vi "move to target point.vi"(2 "PIS Close":bool, 8 "precision of nodes":i32=6, 9 "Litho Speed":dbl=5e-07 format="%#_6pm/s", 10 "Z SetPoint":dbl format="%#_6p", 11 "Target Point\n(  x      ,       y   )":dbl[](array[numeric])=[-5e-06, -5e-06] min=-4.5e-05 max=4.5e-05 step=1e-09 format="%#_6pm") -> ()   [LabVIEW 2013]
uses:
  simulator/Global Variables.vi
  Cypher XY LVDT Parameters.vi
panel:
  in  "?":bool
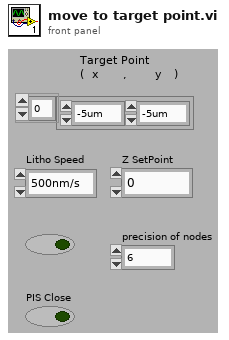
[diagram p1: front panel]
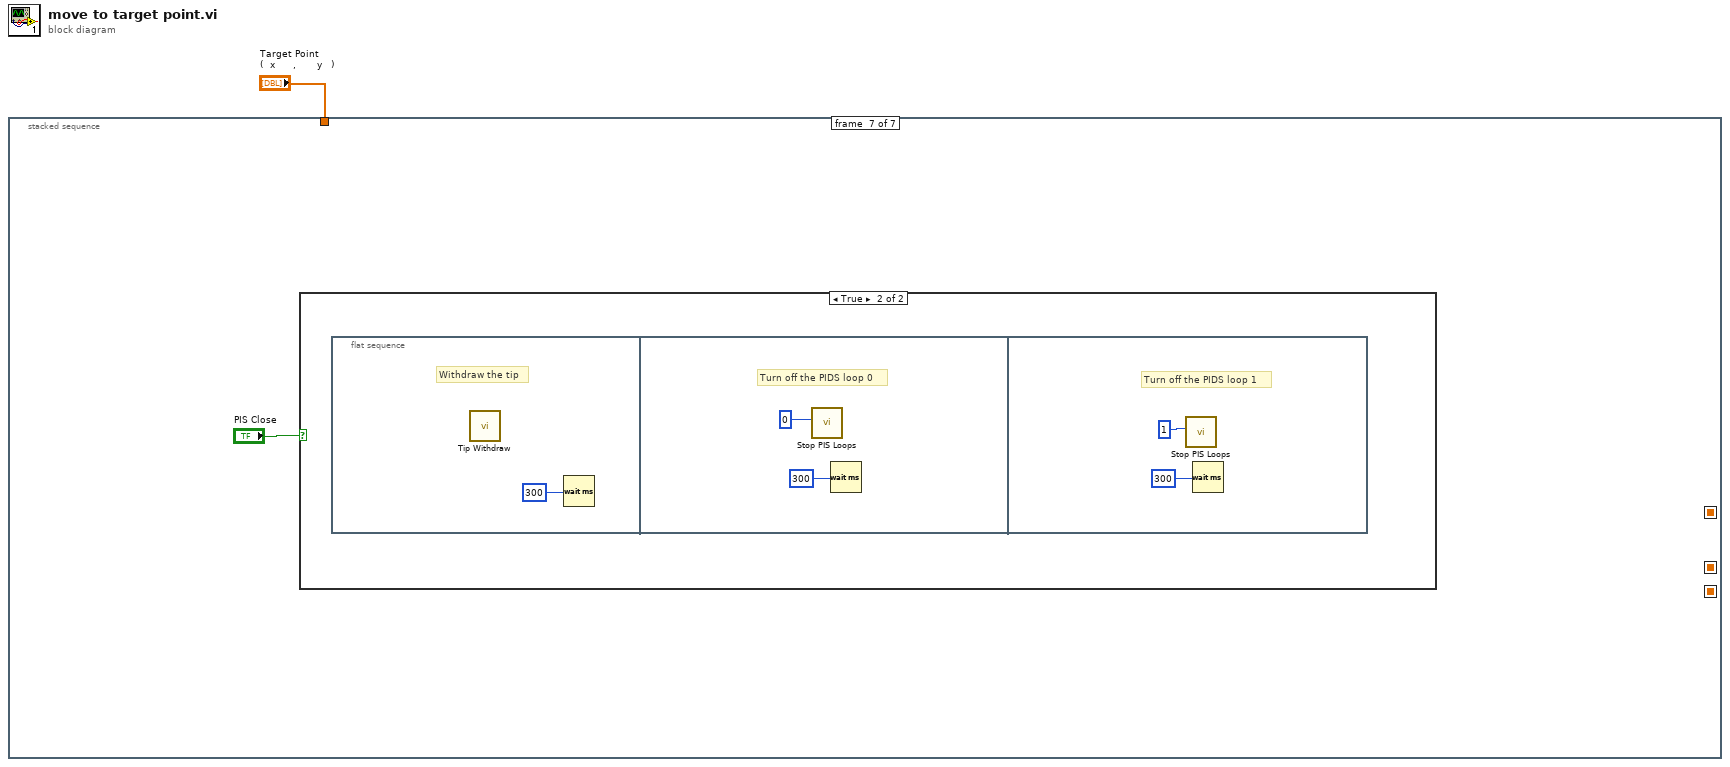
[diagram p0: block diagram]
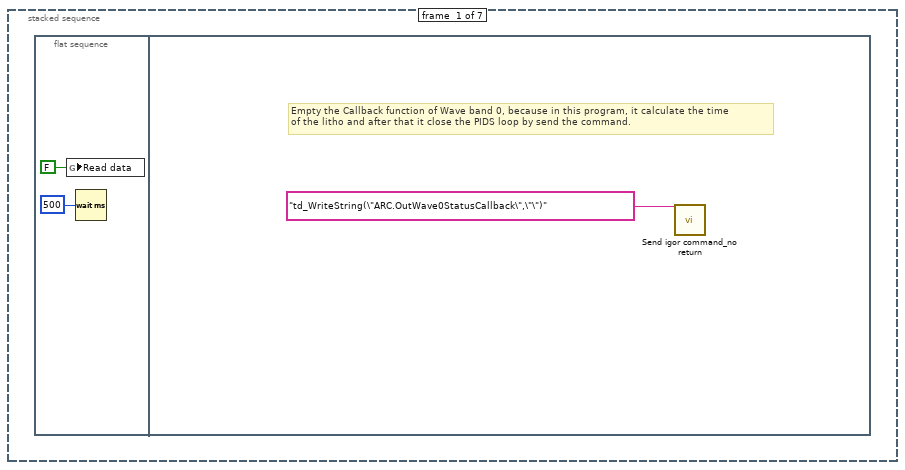
[diagram p2: hidden frame]
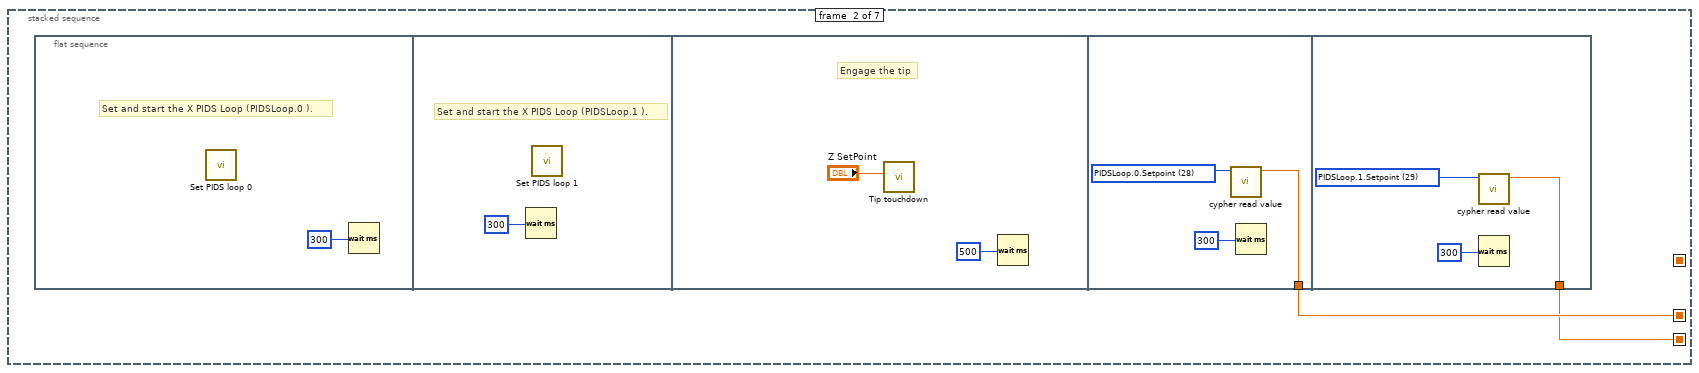
[diagram p3: hidden frame]
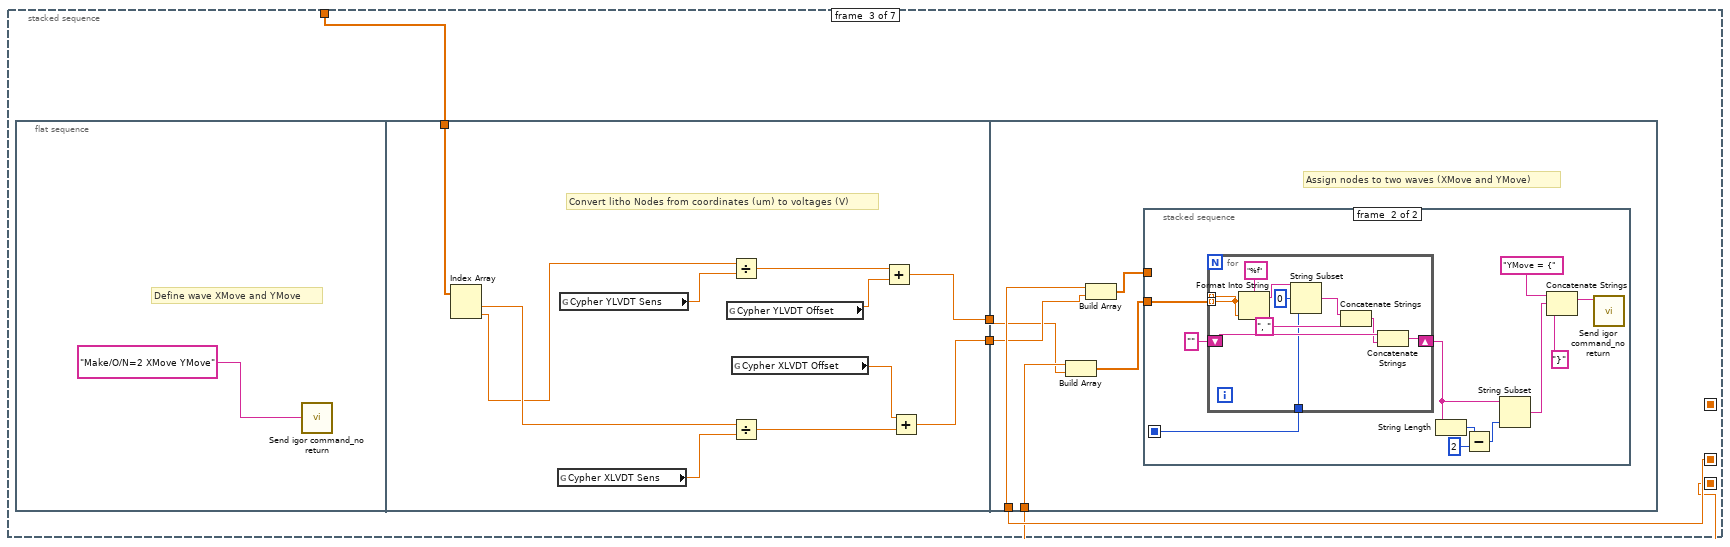
[diagram p4: hidden frame]
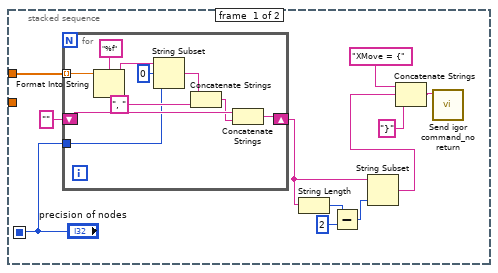
[diagram p5: hidden frame]
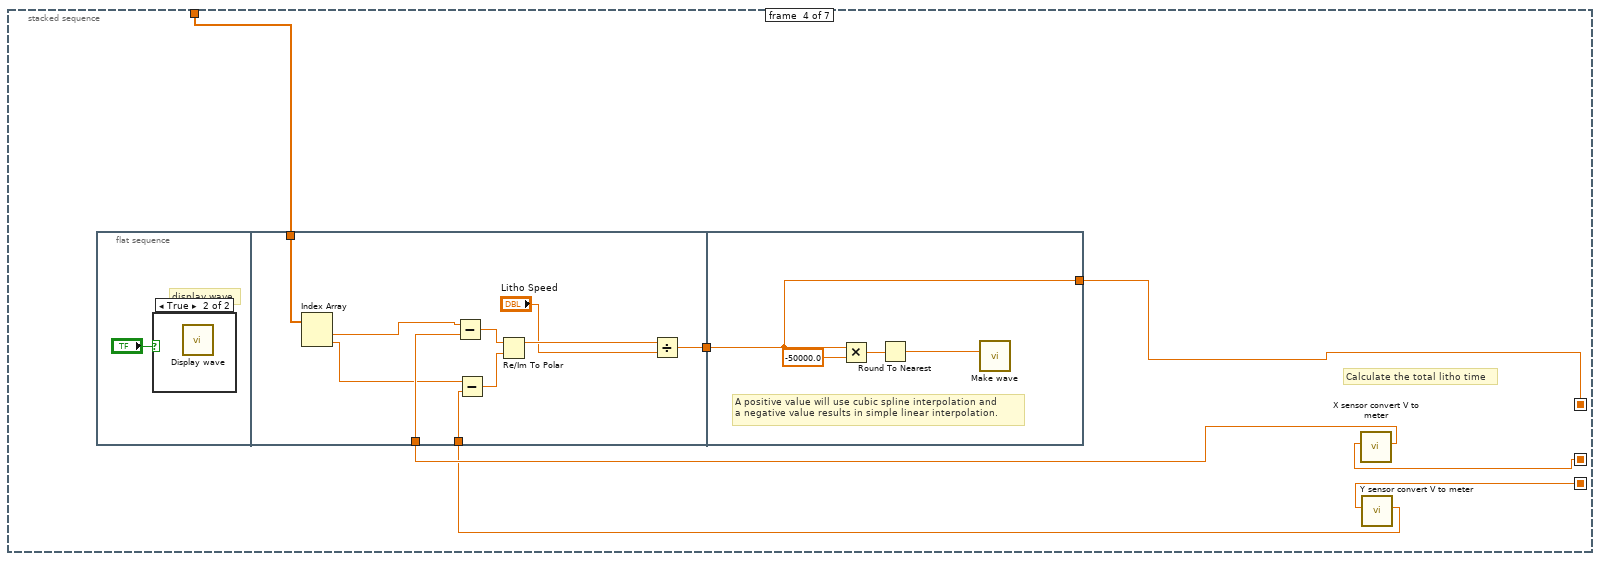
[diagram p6: hidden frame]
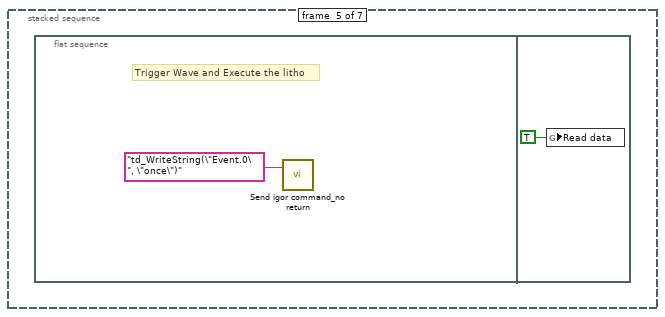
[diagram p8: hidden frame]
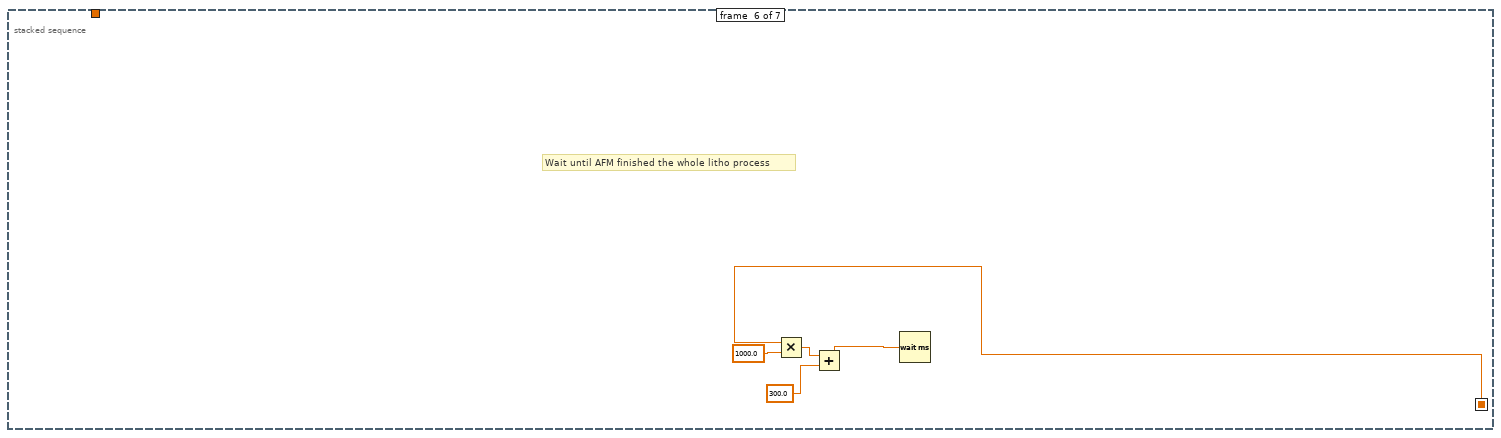
[diagram p9: hidden frame]
diagram:
  n1 = stacked-sequence {
    seq-local: [_ _ _ w87 _ _ _] -> [_ _ _ _ _ w109 _]
    seq-local: [_ w6 _ _ _ _ _] -> [_ _ w18 w86 _ _ _]
    seq-local: [_ w5 _ _ _ _ _] -> [_ _ w17 w85 _ _ _]
    tunnel: "Target Point\n(  x      ,       y   )" -> [_ _ w19 w84 _ _ _]
    frame #0 {
      n2 = flat-sequence {
        frame #0 {
          n3 = global write "Global Variables.vi" "Read data"(FALSE ("Read data")) -> ()
          n4 = Wait (ms)(milliseconds to wait=u32 500) -> ()  [unwired: 1 out]
        }
        frame #1 {
          # "Empty the Callback function of Wave band 0, because in this program, it calculate the time \nof the litho and after that it close the PIDS loop by send the command."
          n5 = call "Send igor command_no return.vi"("Command"="td_WriteString(\"ARC.OutWave0StatusCallback\",\"\")") -> ()  [unwired: 11 out]
        }
      }
    }
    frame #1 {
      n6 = flat-sequence {
        tunnel: [w12] -> w6
        tunnel: [w15] -> w5
        frame #0 {
          # "Set and start the X PIDS Loop (PIDSLoop.0 )."
          n7 = call "Set PIDS loop 0.vi"() -> ()  [unwired: 12 in]
          n8 = Wait (ms)(milliseconds to wait=u32 300) -> ()  [unwired: 1 out]
        }
        frame #1 {
          # "Set and start the X PIDS Loop (PIDSLoop.1 )."
          n9 = Wait (ms)(milliseconds to wait=u32 300) -> ()  [unwired: 1 out]
          n10 = call "Set PIDS loop 1.vi"() -> ()  [unwired: 12 in]
        }
        frame #2 {
          # "Engage the tip"
          n11 = call "Tip touchdown.vi"("Z SetPoint"="Z SetPoint") -> ()  [unwired: 11 out]
          n12 = Wait (ms)(milliseconds to wait=u32 500) -> ()  [unwired: 1 out]
        }
        frame #3 {
          w13 = u16 28 items=["XSensor", "YSensor", "ZSensor", "InA", "InB", "InFast", "In_Amplitude1", "In_Amplitude2", "In_Phase1", "In_Phase2", "PiezoX", "PiezoY", "PiezoZ", "OutA", "OutB", "OutC", "DDS_Frequency1", "DDS_Frequency2", "DDS_Amplitude1", "DDS_Amplitude2", "DDS_DCOffset", "Laser_Sum", "Laser_Difference", "Laser_Lateral", "XLVDT Sensitivity", "YLVDT Sensitivity", "XLVDT Offset", "YLVDT Offset", "PIDSLoop.0.Setpoint", "PIDSLoop.1.Setpoint"] ("Input")
          n13 = call "cypher read value.vi"("Input"=w13) -> ("Result"=w12:dbl)  [unwired: 10 in]
          n14 = Wait (ms)(milliseconds to wait=u32 300) -> ()  [unwired: 1 out]
        }
        frame #4 {
          w16 = u16 29 items=["XSensor", "YSensor", "ZSensor", "InA", "InB", "InFast", "In_Amplitude1", "In_Amplitude2", "In_Phase1", "In_Phase2", "PiezoX", "PiezoY", "PiezoZ", "OutA", "OutB", "OutC", "DDS_Frequency1", "DDS_Frequency2", "DDS_Amplitude1", "DDS_Amplitude2", "DDS_DCOffset", "Laser_Sum", "Laser_Difference", "Laser_Lateral", "XLVDT Sensitivity", "YLVDT Sensitivity", "XLVDT Offset", "YLVDT Offset", "PIDSLoop.0.Setpoint", "PIDSLoop.1.Setpoint"] ("Input")
          n15 = call "cypher read value.vi"("Input"=w16) -> ("Result"=w15:dbl)  [unwired: 10 in]
          n16 = Wait (ms)(milliseconds to wait=u32 300) -> ()  [unwired: 1 out]
        }
      }
    }
    frame #2 {
      n17 = flat-sequence {
        tunnel: [w27] -> w21
        tunnel: [w26] -> w20
        tunnel: w19 -> [w25]
        tunnel: w21 -> [w35]
        tunnel: w20 -> [w37]
        tunnel: w18 -> [w39]
        tunnel: w17 -> [w38]
        frame #0 {
          # "Define wave XMove and YMove"
          n18 = call "Send igor command_no return.vi"("Command"="Make/O/N=2 XMove YMove") -> ()  [unwired: 11 out]
        }
        frame #1 {
          # "Convert litho Nodes from coordinates (um) to voltages (V)"
          n19 = Index Array(array=w25) -> (element #1=w24:dbl, element #2=w23:dbl)  [unwired: 2 in]
          n20 = global read "Cypher XY LVDT Parameters.vi" "Cypher XLVDT Sens"() -> (w30:dbl)
          n21 = global read "Cypher XY LVDT Parameters.vi" "Cypher YLVDT Sens"() -> (w31:dbl)
          n22 = global read "Cypher XY LVDT Parameters.vi" "Cypher YLVDT Offset"() -> (w28:dbl)
          n23 = Divide(x=w23, y=w31) -> (x/y=w32:dbl)
          n24 = Divide(x=w24, y=w30) -> (x/y=w33:dbl)
          n25 = global read "Cypher XY LVDT Parameters.vi" "Cypher XLVDT Offset"() -> (w29:dbl)
          n26 = Add(x=w32, y=w28) -> (x+y=w27:dbl)
          n27 = Add(x=w29, y=w33) -> (x+y=w26:dbl)
        }
        frame #2 {
          # "Assign nodes to two waves (XMove and YMove)"
          n28 = Build Array(w38, w35) -> (w34:dbl[])
          n29 = Build Array(w39, w37) -> (w36:dbl[])
          n30 = stacked-sequence {
            seq-local: ["precision of nodes" _] -> [_ w61]
            tunnel: w36 -> [w48 _]
            tunnel: w34 -> [_ w67]
            frame #0 {
              n31 = for {
                tunnel: w48 -> [w59] mode=indexing
                shift-right: [w57] -> w45
                shift-left: "" -> [w56]
                tunnel: "precision of nodes" -> [w51]
                n32 = Format Into String(format string="%f", w59) -> (resulting string=w53:string)  [unwired: 2 in, 1 out]
                n33 = String Subset(string=w53, offset (0)=0, length (rest)=w51) -> (substring=w52:string)
                n34 = Concatenate Strings(w52, ", " ("string")) -> (w55:string)
                n35 = Concatenate Strings(w56, w55) -> (w57:string)
              }
              n36 = String Length(string=w45) -> (length=w44:i32)
              n37 = Subtract(x=w44, y=2) -> (x-y=w42:i32)
              n38 = String Subset(string=w45, length (rest)=w42) -> (substring=w41:string)  [unwired: 1 in]
              n39 = Concatenate Strings("XMove = {" ("string"), w41, "}" ("string")) -> (w50:string)
              n40 = call "Send igor command_no return.vi"("Command"=w50) -> ()  [unwired: 11 out]
            }
            frame #1 {
              n41 = for {
                tunnel: [w76] -> _ mode=indexing
                shift-right: [w79] -> w62
                shift-left: "" -> [w78]
                tunnel: w67 -> [w76] mode=indexing
                tunnel: w61 -> [w72]
                n42 = Format Into String(format string="%f", w76) -> (resulting string=w75:string)  [unwired: 2 in, 1 out]
                n43 = String Subset(string=w75, offset (0)=0, length (rest)=w72) -> (substring=w73:string)
                n44 = Concatenate Strings(w73, ", " ("string")) -> (w77:string)
                n45 = Concatenate Strings(w78, w77) -> (w79:string)
              }
              n46 = String Length(string=w62) -> (length=w66:i32)
              n47 = Subtract(x=w66, y=2) -> (x-y=w64:i32)
              n48 = String Subset(string=w62, length (rest)=w64) -> (substring=w63:string)  [unwired: 1 in]
              n49 = Concatenate Strings("YMove = {" ("string"), w63, "}" ("string")) -> (w68:string)
              n50 = call "Send igor command_no return.vi"("Command"=w68) -> ()  [unwired: 11 out]
            }
          }
        }
      }
    }
    frame #3 {
      # "Calculate the total litho time"
      n51 = flat-sequence {
        tunnel: [w95] -> w88
        tunnel: w84 -> [w94]
        tunnel: w83 -> [w92]
        tunnel: w82 -> [w90]
        tunnel: w88 -> [w100]
        tunnel: [w100] -> w87
        frame #0 {
          # "display wave"
          n52 = case shown="True" "?" {
            frame False {
            }
            frame True {
              n53 = call "Display wave.vi"() -> ()  [unwired: 1 out]
            }
          }
        }
        frame #1 {
          n54 = Index Array(array=w94) -> (element #1=w93:dbl, element #2=w91:dbl)  [unwired: 2 in]
          n55 = Subtract(x=w93, y=w92) -> (x-y=w99:dbl)
          n56 = Subtract(x=w91, y=w90) -> (x-y=w98:dbl)
          n57 = Re/Im To Polar(2:w98, 3:w99) -> (1:w97:dbl)  [unwired: 1 out]
          n58 = Divide(x=w97, y="Litho Speed") -> (x/y=w95:dbl)
        }
        frame #2 {
          # "A positive value will use cubic spline interpolation and \na negative value results in simple linear interpolation."
          n59 = Multiply(x=w100, y=-50000.0) -> (x*y=w102:dbl)
          n60 = Round To Nearest(number=w102) -> (nearest integer value=w101:dbl)
          n61 = call "Make wave.vi"("Totalpoints"=w101) -> ()  [unwired: 11 out]
        }
      }
      n62 = call "X sensor convert V to meter.vi"("Sensor X Voltage"=w86) -> ("X coordinate"=w83:dbl)  [unwired: 10 in]
      n63 = call "Y sensor convert V to meter.vi"("Sensor Y Voltage"=w85) -> ("Y coordinate"=w82:dbl)  [unwired: 10 in]
    }
    frame #4 {
      n64 = flat-sequence {
        frame #0 {
          # "Trigger Wave and Execute the litho"
          n65 = call "Send igor command_no return.vi"("Command"="td_WriteString(\"Event.0\", \"once\")") -> ()  [unwired: 11 out]
        }
        frame #1 {
          n66 = global write "Global Variables.vi" "Read data"(TRUE ("Read data")) -> ()
        }
      }
    }
    frame #5 {
      # "Wait until AFM finished the whole litho process"
      n67 = Multiply(x=w109, y=1000.0) -> (x*y=w108:dbl)
      n68 = Add(x=w108, y=300.0) -> (x+y=w106:dbl)
      n69 = Wait (ms)(milliseconds to wait=w106) -> ()  [unwired: 1 out]
    }
    frame #6 {
      n70 = case shown="True" "PIS Close" {
        frame False {
        }
        frame True {
          n71 = flat-sequence {
            frame #0 {
              # "Withdraw the tip"
              n72 = call "Tip Withdraw.vi"() -> ()  [unwired: 1 in]
              n73 = Wait (ms)(milliseconds to wait=u32 300) -> ()  [unwired: 1 out]
            }
            frame #1 {
              # "Turn off the PIDS loop 0"
              n74 = call "Stop PIS Loops.vi"("PIS Loop Number (0-5)"=u32 0) -> ()  [unwired: 11 out]
              n75 = Wait (ms)(milliseconds to wait=u32 300) -> ()  [unwired: 1 out]
            }
            frame #2 {
              # "Turn off the PIDS loop 1"
              n76 = call "Stop PIS Loops.vi"("PIS Loop Number (0-5)"=u32 1) -> ()  [unwired: 11 out]
              n77 = Wait (ms)(milliseconds to wait=u32 300) -> ()  [unwired: 1 out]
            }
          }
        }
      }
    }
  }
